vi "GetDataType.vi"(0 "object in":refnum<class "Client.lvclass">, 5 "Error In":errorcluster) -> (14 "object out":refnum<class "Client.lvclass">, 15 "Data Type":refnum<class "DataType.lvclass">, 19 "Error Out":errorcluster)   [LabVIEW 2024, in "Client.lvclass"]
uses:
  <resource>/Framework/Providers/Open_GDS/ClassProviders/Provider_LvNativeClass/Templates/NativeBaseTemplate/NativeBaseTemplate.lvclass/NativeBaseTemplate.ctl
  Client.lvclass
  Client.lvclass/Client.ctl
  Abstractions/DataType/DataType.lvclass
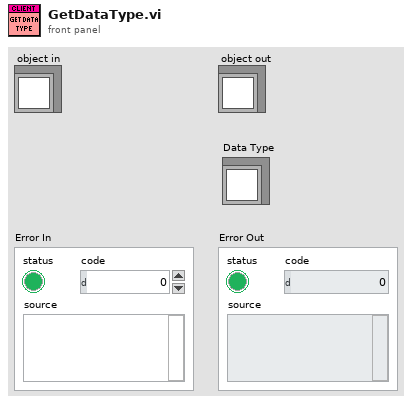
[diagram p1: front panel]
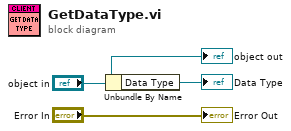
[diagram p0: block diagram]
diagram:
  n1 = Unbundle By Name("object in") -> ("Data Type"=→"Data Type":refnum<class "DataType.lvclass">)
  "Error Out" <- "Error In"
  "object out" <- "object in"
